vi "Periodic Tasks.vi"() -> ()   [LabVIEW 2012]
doc: "This VI runs in parallel to other tasks. It can contain as many user-defined periodic loops as you need. These can carry out PID or other sorts of timed response."
uses:
  <vilib>/Rock Robotics/SystemInterfaces/Utilities/FPGA_UtilitiesLED Source.ctl
  <vilib>/Rock Robotics/SystemInterfaces/Utilities/FPGA_UtilitiesLED State.ctl
  Robot Global Data.vi
panel:
  out "Left Drive":dbl
  out "Right Drive":dbl
  in  "Lateral Constant":dbl=0.5
  in  "Shoot Deadband":dbl=0.1
  in  "In Cluster":T1
  out "Angular Rate":dbl
  out "Angle":dbl
  out "Rate":dbl
  out "Direction":bool
  out "Distance":dbl
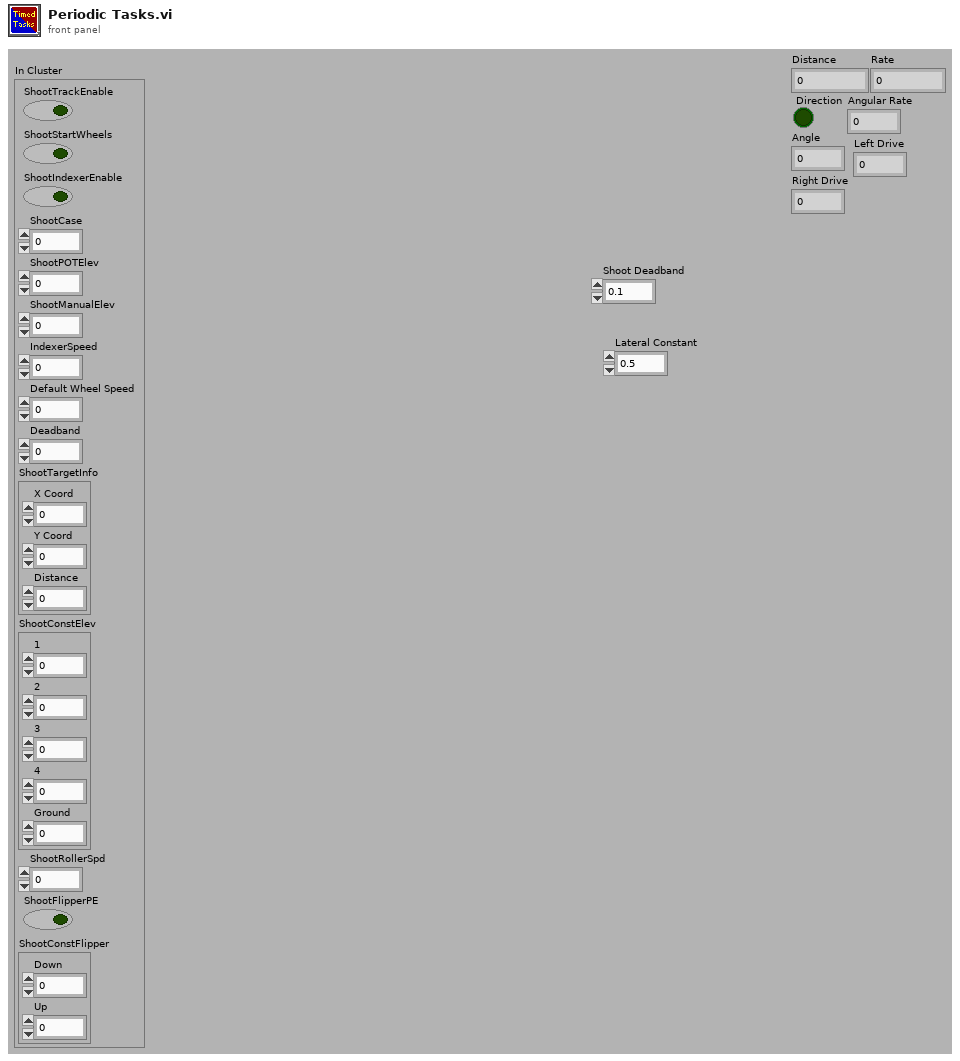
[diagram p1: front panel]
types:
  T1 = cluster{"ShootTrackEnable":bool, "ShootStartWheels":bool, "ShootIndexerEnable":bool, "ShootCase":dbl, "ShootPOTElev":dbl, "ShootManualElev":dbl, "IndexerSpeed":dbl, "Default Wheel Speed":dbl, "Deadband":dbl, "ShootTargetInfo":cluster{"X Coord":dbl, "Y Coord":dbl, "Distance":dbl}, "ShootConstElev":cluster{"1":dbl, "2":dbl, "3":dbl, "4":dbl, "Ground":dbl}, "ShootRollerSpd":dbl, "ShootFlipperPE":bool, "ShootConstFlipper":cluster{"Down":dbl, "Up":dbl}}
  T2 = typedef "FPGA_UtilitiesLED State.ctl" = enum16{"Off", "On", "Toggle"}
  T3 = typedef "FPGA_UtilitiesLED Source.ctl" = enum16{"User LED", "FPGA LED"}
  T4 = typedef "WPI_GyroDevRef.ctl" = cluster{"DevStatus":errorcluster, "Analog Module":T5, "Analog Channel":T6, "Offset":dbl, "Gain (VoltsPerDegree/Second)":dbl}
  T5 = typedef "FPGA_TypedefAnalogModule.ctl" = enum16{"Analog Module 1", "Analog Module 2"}
  T6 = typedef "FPGA_AIChannel.ctl" = enum8{"AI 1", "AI 2", "AI 3", "AI 4", "AI 5", "AI 6", "AI 7", "AI 8", "Invalid"}
  T7 = typedef "WPI_EncoderDevRef.ctl" = cluster{"DevStatus":errorcluster, "EncoderIndex":T8, "CounterIndex":T9, "DistancePerCount":dbl, "Decoding Type":T10}
  T8 = typedef "FPGA_EncoderIdx.ctl" = enum8{"Enc 0", "Enc 1", "Enc 2", "Enc 3", "Invalid"}
  T9 = typedef "FPGA_CounterCtrSystemIndex.ctl" = enum8{"Ctr 0", "Ctr 1", "Ctr 2", "Ctr 3", "Ctr 4", "Ctr 5", "Ctr 6", "Ctr 7", "Invalid"}
  T10 = typedef "WPI_EncoderType.ctl" = enum16{"1x", "2x", "4x"}
  T11 = typedef "WPI_DigitalInputDevRef.ctl" = cluster{"DevStatus":errorcluster, "DIO Channel":T12, "Digital Module":T13}
  T12 = typedef "FPGA_DIOChannel.ctl" = enum8{"DIO 1", "DIO 2", "DIO 3", "DIO 4", "DIO 5", "DIO 6", "DIO 7", "DIO 8", "DIO 9", "DIO 10", "DIO 11", "DIO 12", "DIO 13", "DIO 14", "Invalid"}
  T13 = typedef "FPGA_TypedefDigitalModule.ctl" = enum16{"Digital Module 1", "Digital Module 2"}
  T14 = typedef "WPI_AnalogChannelDevRef.ctl" = cluster{"DevStatus":errorcluster, "Analog Module":T5, "Analog Channel":T6}
  T15 = cluster{"Ground":dbl, "1":dbl, "2":dbl, "3":dbl, "4":dbl}
  T16 = cluster{"ShootOutIndexer":dbl, "ShootOutElev":dbl, "ShootOutCase":dbl, "ShootOutWheelF":dbl, "ShootOutRollers":dbl, "ShootOutFlipper":dbl}
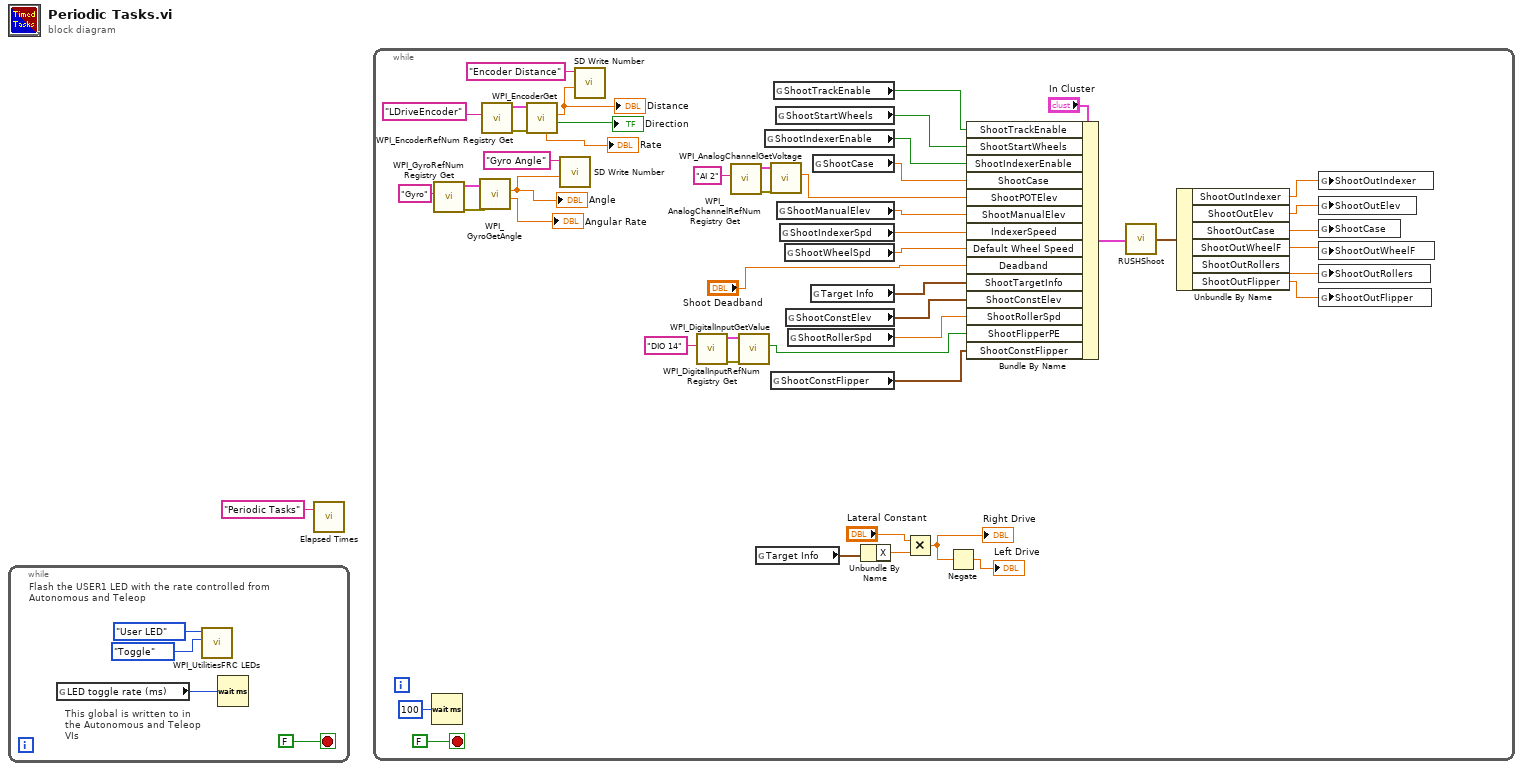
[diagram p0: block diagram]
diagram:
  n1 = while {
    stop <- FALSE stop-if-true
    # "This global is written to in the Autonomous and Teleop VIs"
    # "Flash the USER1 LED with the rate controlled from Autonomous and Teleop"
    n2 = global read "Robot Global Data.vi" "LED toggle rate (ms)"() -> (w2:u32)
    n3 = call <vilib>:"WPI_UtilitiesFRC LEDs.vi"("State"=FPGA_UtilitiesLED_State."Toggle", "LED Type"=FPGA_UtilitiesLED_Source."User LED") -> ()  [unwired: 1 in, 9 out]
    n4 = Wait (ms)(milliseconds to wait=w2) -> ()  [unwired: 1 out]
  }
  n5 = call "Elapsed Times.vi"("Call Name"="Periodic Tasks") -> ()  [unwired: 2 in, 1 out]
  n6 = while {
    stop <- FALSE stop-if-true
    n7 = Wait (ms)(milliseconds to wait=u32 100) -> ()  [unwired: 1 out]
    n8 = call <vilib>:"WPI_GyroRefNum Registry Get.vi"("refnum name"="Gyro") -> ("error out"=w50:errorcluster, "GyroDevRef"=w49:T4)  [unwired: 9 in]
    n9 = call <vilib>:"WPI_GyroGetAngle.vi"("error in (no error)"=w50, "GyroDevRef"=w49) -> ("Angular Rate"=→"Angular Rate":dbl, "Angle"=w41:dbl)  [unwired: 6 in, 2 out]
    "Angle" <- w41
    n10 = call <vilib>:"WPI_EncoderRefNum Registry Get.vi"("refnum name"="LDriveEncoder") -> ("error out"=w52:errorcluster, "EncoderDevRef"=w51:T7)  [unwired: 9 in]
    n11 = call <vilib>:"WPI_EncoderGet.vi"("error in (no error)"=w52, "EncoderDevRef"=w51) -> ("Direction"=→"Direction":bool, "Distance"=w40:dbl, "Rate"=→"Rate":dbl)  [unwired: 4 in, 3 out]
    "Distance" <- w40
    n12 = call <vilib>:"SD Write Number.vi"("Numeric"=w41, "Name"="Gyro Angle") -> ()  [unwired: 8 in, 2 out]
    n13 = call <vilib>:"SD Write Number.vi"("Numeric"=w40, "Name"="Encoder Distance") -> ()  [unwired: 8 in, 2 out]
    n14 = call <vilib>:"WPI_DigitalInputRefNum Registry Get.vi"("refnum name"="DIO 14") -> ("error out"=w15:errorcluster, "DigitalInputDevRef"=w14:T11)  [unwired: 9 in]
    n15 = call <vilib>:"WPI_AnalogChannelRefNum Registry Get.vi"("refnum name"="AI 2") -> ("error out"=w18:errorcluster, "AIDeviceRef"=w17:T14)  [unwired: 9 in]
    n16 = call <vilib>:"WPI_DigitalInputGetValue.vi"("error in (no error)"=w15, "DigitalInputDevRef"=w14) -> ("Value"=w12:bool)  [unwired: 7 in, 2 out]
    n17 = global read "Robot Global Data.vi" "Target Info"() -> (w8:cluster{"X":dbl, "Y":dbl, "Distance (ft)":dbl})
    n18 = global read "Robot Global Data.vi" "ShootIndexerEnable"() -> (w29:bool)
    n19 = call <vilib>:"WPI_AnalogChannelGetVoltage.vi"("error in (no error)"=w18, "AIDeviceRef"=w17) -> ("Voltage"=w16:dbl)  [unwired: 7 in, 2 out]
    n20 = global read "Robot Global Data.vi" "ShootConstFlipper"() -> (w34:cluster{"Down":dbl, "Up":dbl})
    n21 = global read "Robot Global Data.vi" "ShootTrackEnable"() -> (w31:bool)
    n22 = global read "Robot Global Data.vi" "ShootStartWheels"() -> (w30:bool)
    n23 = global read "Robot Global Data.vi" "ShootManualElev"() -> (w28:dbl)
    n24 = global read "Robot Global Data.vi" "ShootIndexerSpd"() -> (w38:dbl)
    n25 = global read "Robot Global Data.vi" "ShootWheelSpd"() -> (w37:dbl)
    n26 = global read "Robot Global Data.vi" "ShootConstElev"() -> (w35:T15)
    n27 = global read "Robot Global Data.vi" "ShootRollerSpd"() -> (w27:dbl)
    n28 = global read "Robot Global Data.vi" "Target Info"() -> (w36:cluster{"X":dbl, "Y":dbl, "Distance (ft)":dbl})
    n29 = global read "Robot Global Data.vi" "ShootCase"() -> (w39:dbl)
    n30 = Unbundle By Name(w8) -> ("X"=w10:dbl)
    n31 = Multiply(x="Lateral Constant", y=w10) -> (x*y=w7:dbl)
    "Right Drive" <- w7
    n32 = Negate(x=w7) -> (-x=→"Left Drive":dbl)
    n33 = Bundle By Name(cluster="In Cluster", "ShootTrackEnable"=w31, "ShootStartWheels"=w30, "ShootIndexerEnable"=w29, "ShootCase"=w39, "ShootPOTElev"=w16, "ShootManualElev"=w28, "IndexerSpeed"=w38, "Default Wheel Speed"=w37, "Deadband"="Shoot Deadband", "ShootTargetInfo"=w36, "ShootConstElev"=w35, "ShootRollerSpd"=w27, "ShootFlipperPE"=w12, "ShootConstFlipper"=w34) -> (w32:T1)
    n34 = call "RUSHShoot.vi"("In Cluster"=w32) -> ("Out Cluster"=w26:T16)
    n35 = Unbundle By Name(w26) -> ("ShootOutIndexer"=w23:dbl, "ShootOutElev"=w24:dbl, "ShootOutCase"=w25:dbl, "ShootOutWheelF"=w22:dbl, "ShootOutRollers"=w21:dbl, "ShootOutFlipper"=w20:dbl)
    n36 = global write "Robot Global Data.vi" "ShootOutIndexer"(w23) -> ()
    n37 = global write "Robot Global Data.vi" "ShootOutElev"(w24) -> ()
    n38 = global write "Robot Global Data.vi" "ShootCase"(w25) -> ()
    n39 = global write "Robot Global Data.vi" "ShootOutWheelF"(w22) -> ()
    n40 = global write "Robot Global Data.vi" "ShootOutRollers"(w21) -> ()
    n41 = global write "Robot Global Data.vi" "ShootOutFlipper"(w20) -> ()
  }
